vi "SetJogParameters.vi"(8 "error in (no error)":errorcluster, 9 "Jog Parameters":T1, 10 "channel":i32(ring)=1 items=["Channel1"=1, "Channel2"=2, "Channel3"=3, "Channel4"=4], 11 "KIM Reference":refnum<k24>) -> (0 "error out":errorcluster, 3 "KIM Reference":refnum<k24>)   [LabVIEW 2023, in "KIM101.lvlib"]
uses:
  KIM101/KIM101.lvlib
  C:/Users/quantum/Documents/LVDAQ/UIs/TranslationStage_UI/Thorlabs.MotionControl.KCube.InertialMotorCLI.dll
  UIs/TranslationStage_UI/Thorlabs.MotionControl.KCube.InertialMotorCLI.dll
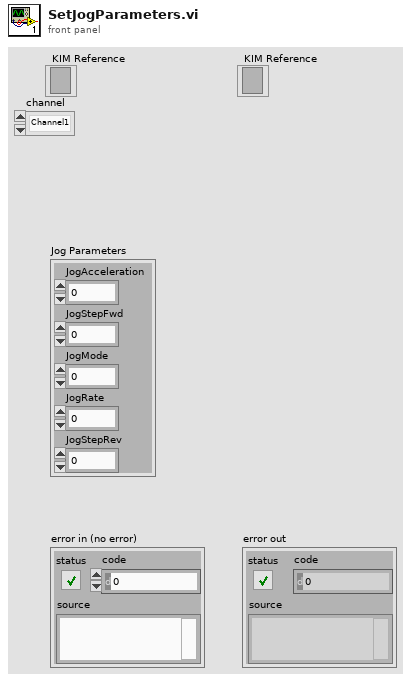
[diagram p1: front panel]
types:
  T1 = cluster{"JogAcceleration":i32, "JogStepFwd":i32, "JogMode":i32, "JogRate":i32, "JogStepRev":i32}
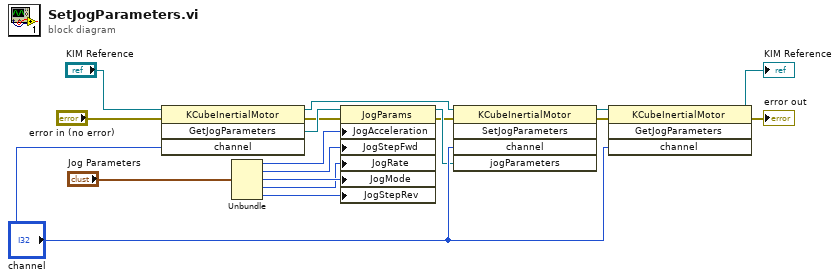
[diagram p0: block diagram]
diagram:
  n1 = invoke class="KCubeInertialMotor" method="GetJogParameters"(reference="KIM Reference", error in="error in (no error)", "channel"="channel") -> (reference out=w15:refnum<k24>, error out=w5:errorcluster, "GetJogParameters"=w12:refnum<k24>)  [unwired: 1 in, 1 out]
  n2 = Unbundle("Jog Parameters") -> ("JogAcceleration"=w8:i32, "JogStepFwd"=w17:i32, "JogMode"=w18:i32, "JogRate"=w7:i32, "JogStepRev"=w6:i32)
  n3 = property class="JogParams"(reference=w12, error in=w5, "JogAcceleration"=w8, "JogStepFwd"=w17, "JogRate"=w7, "JogMode"=w18, "JogStepRev"=w6) -> (reference out=w11:refnum<k24>, error out=w4:errorcluster)
  n4 = invoke class="KCubeInertialMotor" method="SetJogParameters"(reference=w15, error in=w4, "channel"="channel", "jogParameters"=w11) -> (reference out=w10:refnum<k24>, error out=w3:errorcluster)  [unwired: 1 in, 3 out]
  n5 = invoke class="KCubeInertialMotor" method="GetJogParameters"(reference=w10, error in=w3, "channel"="channel") -> (reference out=→"KIM Reference":refnum<k24>, error out=→"error out":errorcluster)  [unwired: 1 in, 2 out]
